vi "Stop.vi"(6 "timeout in ms (-1)":i32=-1, 8 "error in (no error)":errorcluster, 11 "JKI SMO in":refnum<class "JKI SMO.lvclass">) -> (0 "error out":errorcluster, 3 "JKI SMO out":refnum<class "JKI SMO.lvclass">)   [LabVIEW 2013, in "JKI SMO.lvclass"]
doc: "This method signal all the running processes to shutdown.\n\n<b>ms timeout</b> is the max amount of time allowed for the process to shutdown before an error is reported. <b>ms timeout</b> default is -1 = never times out\n\nNote 01: This method is overridable by descendant\nNote 02: When overridden, Call Parent Method is required\n\n---------------------------------------------------------------\nJKI State Machine Objects™\nhttp://jki.net/state-machine-objects/\nCopyright (C) 2005-2015, JKI <info@jki.net>\nALL RIGHTS RESERVED"
uses:
  JKI SMO.lvclass
panel:
  # "For instructions on how to use the JKI State Machine Objects, examples and video tutorials, visit:\nhttp://jki.net/state-machine-objects/\n\nJKI State Machine Objects™\nhttp://jki.net/state-machine-objects/\nCopyright (C) 2005-2015, JKI <info@jki.net>\nALL RIGHTS RESERVED"
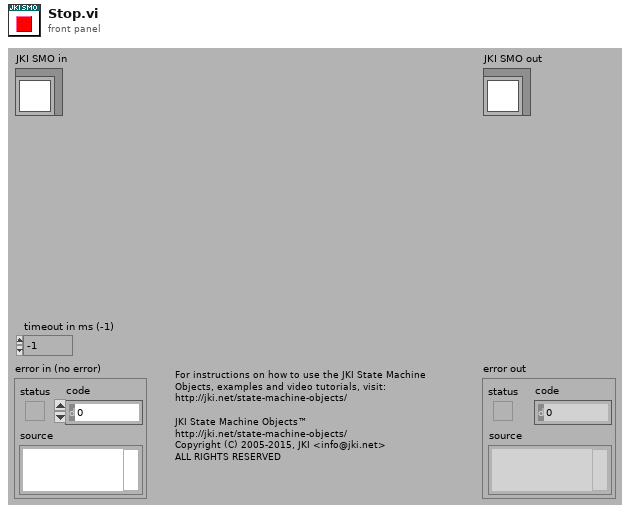
[diagram p1: front panel]
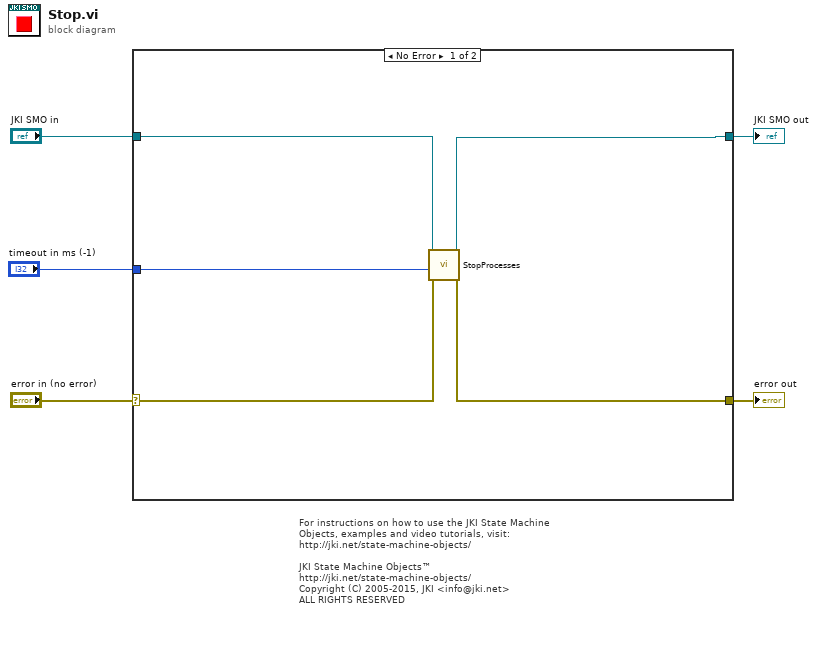
[diagram p0: block diagram]
diagram:
  # "For instructions on how to use the JKI State Machine Objects, examples and video tutorials, visit:\nhttp://jki.net/state-machine-objects/\n\nJKI State Machine Objects™\nhttp://jki.net/state-machine-objects/\nCopyright (C) 2005-2015, JKI <info@jki.net>\nALL RIGHTS RESERVED"
  n1 = case shown="No Error" "error in (no error)" {
    selector: "error in (no error)" -> [w9 w12]
    tunnel: [w8 w12] -> w4
    tunnel: [w7 w11] -> w2
    tunnel: "JKI SMO in" -> [w10 w11]
    tunnel: "timeout in ms (-1)" -> [w6 _]
    frame No Error {
      n2 = call "StopProcesses.vi"("error in (no error)"=w9, "timeout in ms (-1)"=w6, "JKI SMO in"=w10) -> ("error out"=w8:errorcluster, "JKI SMO out"=w7:refnum<class "JKI SMO.lvclass">)  [unwired: 7 in]
    }
    frame Error {
    }
  }
  "error out" <- w4
  "JKI SMO out" <- w2
